vi "Add Fit To Record.vi"(1 "Fit Name":string, 2 "Chain Fit":T2, 3 "Input State":T1=[{"Base Directory"=path "", "Experimental Data"={"Experimental Data"={"Extension (nm)"=[], "Force (pN)"=[], "Name"=""}, "Enabled"=FALSE}, "Chain Fit"={"Experimental Data"={"Extension (nm)"=[], "Force (pN)"=[], "Name"=""}, "Enabled"=FALSE}, "Selected"=FALSE, "Ramp Rate (nm/s)"=0.0, "Spring Constant (pN/nm)"=0.0, "Slope (nm/V)"=0.0}]) -> (0 "State With Fit":T1)   [LabVIEW 2013]
uses:
  Analysis Data.ctl
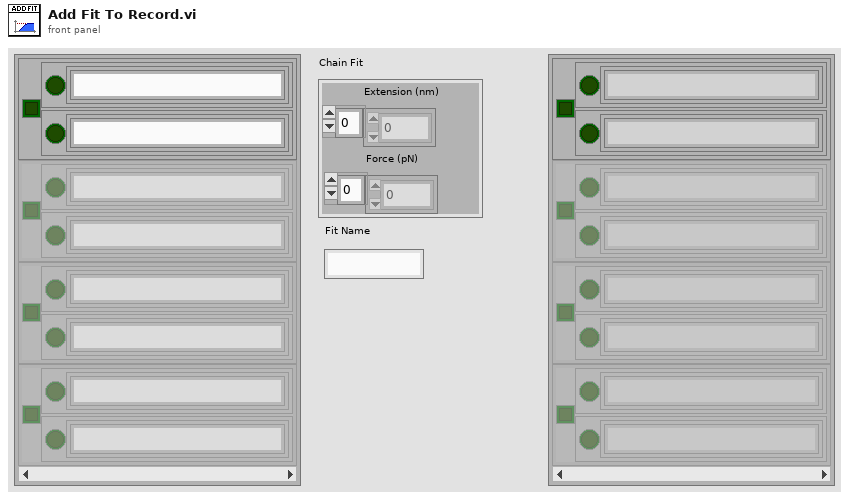
[diagram p1: front panel]
types:
  T1 = typedef "Analysis Data.ctl" = cluster{"Base Directory":path, "Experimental Data":cluster{"Experimental Data":cluster{"Extension (nm)":dbl[], "Force (pN)":dbl[], "Name":string}, "Enabled":bool}, "Chain Fit":cluster{"Experimental Data":cluster{"Extension (nm)":dbl[], "Force (pN)":dbl[], "Name":string}, "Enabled":bool}, "Selected":bool, "Ramp Rate (nm/s)":dbl, "Spring Constant (pN/nm)":dbl, "Slope (nm/V)":dbl}[]
  T2 = cluster{"Extension (nm)":dbl[], "Force (pN)":dbl[]}
  T3 = cluster{"Experimental Data":cluster{"Extension (nm)":dbl[], "Force (pN)":dbl[], "Name":string}, "Enabled":bool}
  T4 = cluster{"Extension (nm)":dbl[], "Force (pN)":dbl[], "Name":string}
  T5 = cluster{"Base Directory":path, "Experimental Data":cluster{"Experimental Data":cluster{"Extension (nm)":dbl[], "Force (pN)":dbl[], "Name":string}, "Enabled":bool}, "Chain Fit":cluster{"Experimental Data":cluster{"Extension (nm)":dbl[], "Force (pN)":dbl[], "Name":string}, "Enabled":bool}, "Selected":bool, "Ramp Rate (nm/s)":dbl, "Spring Constant (pN/nm)":dbl, "Slope (nm/V)":dbl}
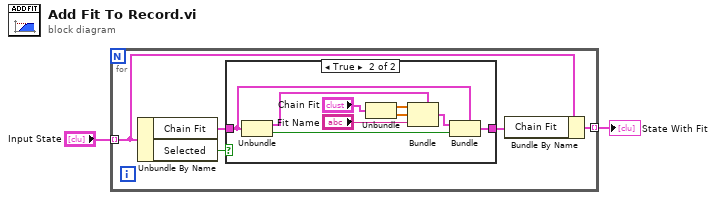
[diagram p0: block diagram]
diagram:
  n1 = for {
    tunnel: "Input State" -> [w5] mode=indexing
    tunnel: [w3] -> w1 mode=indexing
    n2 = Unbundle By Name(w5) -> ("Chain Fit"=w7:T3, "Selected"=w6:bool)
    n3 = case shown="True" w6 {
      tunnel: [w8 w12] -> w4
      tunnel: w7 -> [w8 w9]
      frame False {
      }
      frame True {
        n4 = Unbundle(w9) -> ("Experimental Data"=w10:T4, "Enabled"=w13:bool)
        n5 = Unbundle("Chain Fit") -> ("Extension (nm)"=w15:dbl[], "Force (pN)"=w16:dbl[])
        n6 = Bundle(cluster=w10, "Extension (nm)"=w15, "Force (pN)"=w16, "Name"="Fit Name") -> (w14:T4)
        n7 = Bundle(cluster=w9, "Experimental Data"=w14, "Enabled"=w13) -> (w12:T3)
      }
    }
    n8 = Bundle By Name(cluster=w5, "Chain Fit"=w4) -> (w3:T5)
  }
  "State With Fit" <- w1
